vi "Draw Rect Parabolic Gradient.vi"(7 "Position":cluster{"Left":i16, "Top":i16}, 9 "Percentage(30)":dbl=30.0 format="%0.2f", 10 "Color":u32(colorbox), 11 "Size":cluster{"Width":i16, "Height":i16}) -> (3 "2D Picture":picture)   [LabVIEW 2016, in "Gradient Rectangle.lvclass"]
uses:
  Gradient Rectangle.lvclass
  <vilib>/Analysis/polynomials.llb/Scalar Polynomial Evaluation (DBL).vi
  <vilib>/Analysis/NI_AALPro.lvlib
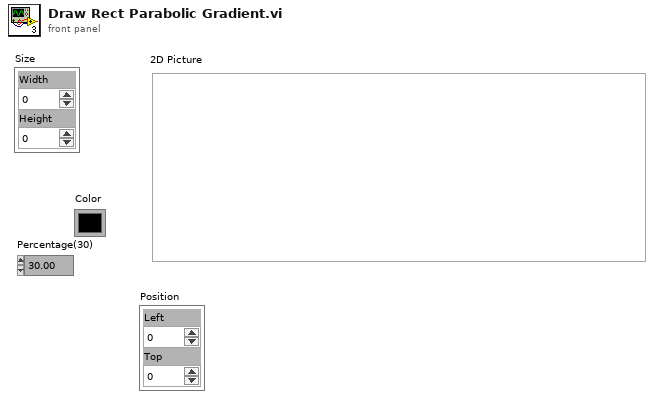
[diagram p1: front panel]
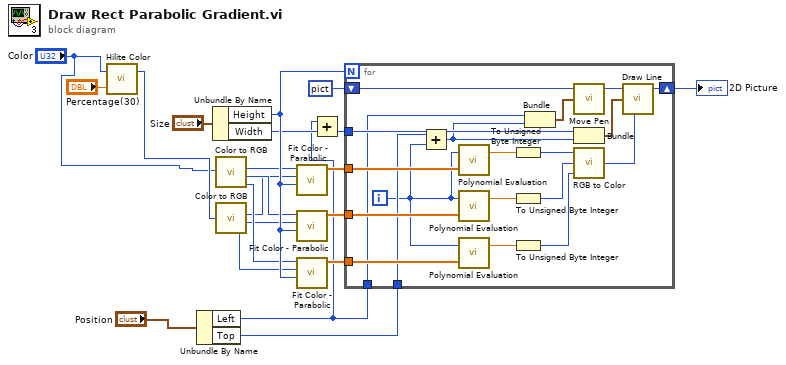
[diagram p0: block diagram]
diagram:
  n1 = call <vilib>:"Hilite Color.vi"("Percentage(30)"="Percentage(30)", "Color In"="Color") -> ("Hilite"=w6:u32)  [unwired: 1 out]
  n2 = Unbundle By Name("Position") -> ("Left"=w1:i16, "Top"=w3:i16)
  n3 = Unbundle By Name("Size") -> ("Height"=w21:i16, "Width"=w20:i16)
  n4 = call <vilib>:"Color to RGB.vi"("Color"="Color") -> ("R"=w12:u8, "G"=w15:u8, "B"=w16:u8)  [unwired: 1 out]
  n5 = call <vilib>:"Color to RGB.vi"("Color"=w6) -> ("R"=w13:u8, "G"=w14:u8, "B"=w17:u8)  [unwired: 1 out]
  n6 = call "Fit Color - Parabolic.vi"("Height"=w21, "Color Shadow"=w13, "Color Hilite"=w12) -> ("Polynomial Coefficients"=w11:dbl[])  [unwired: 8 in]
  n7 = call "Fit Color - Parabolic.vi"("Height"=w21, "Color Shadow"=w14, "Color Hilite"=w15) -> ("Polynomial Coefficients"=w18:dbl[])  [unwired: 8 in]
  n8 = call "Fit Color - Parabolic.vi"("Height"=w21, "Color Shadow"=w17, "Color Hilite"=w16) -> ("Polynomial Coefficients"=w19:dbl[])  [unwired: 8 in]
  n9 = Add(x=w1, y=w20) -> (x+y=w2:i16)
  n10 = for {
    N: w21 -> [_]
    shift-right: [w34] -> w8
    shift-left: picture data[5B] ("new picture") -> [w36]
    tunnel: w11 -> [w41]
    tunnel: w2 -> [w38]
    tunnel: w18 -> [w33]
    tunnel: w19 -> [w32]
    tunnel: w1 -> [w25]
    tunnel: w3 -> [w23]
    i -> [w22]
    n11 = Add(x=w23, y=w22) -> (x+y=w24:i32)
    n12 = call-poly <vilib>:"Polynomial Evaluation.vi"("P(x)"=w41, "a"=w22) -> ("P(a)"=w40:dbl)  [unwired: 1 out]
    n13 = call-poly <vilib>:"Polynomial Evaluation.vi"("P(x)"=w33, "a"=w22) -> ("P(a)"=w30:dbl)  [unwired: 1 out]
    n14 = call-poly <vilib>:"Polynomial Evaluation.vi"("P(x)"=w32, "a"=w22) -> ("P(a)"=w27:dbl)  [unwired: 1 out]
    n15 = To Unsigned Byte Integer(number=w40) -> (unsigned 8bit integer=w31:u8)
    n16 = To Unsigned Byte Integer(number=w30) -> (unsigned 8bit integer=w29:u8)
    n17 = To Unsigned Byte Integer(number=w27) -> (unsigned 8bit integer=w28:u8)
    n18 = Bundle("Left"=w25, w24) -> (w35:cluster{"Left":i16, i32})  [unwired: 1 in]
    n19 = call <vilib>:"Move Pen.vi"("new position"=w35, "picture"=w36) -> ("new picture"=w37:picture)  [unwired: 3 in]
    n20 = Bundle(w38, w24) -> (w39:cluster{i16, i32})  [unwired: 1 in]
    n21 = call <vilib>:"RGB to Color.vi"("B"=w28, "G"=w29, "R"=w31) -> ("Color"=w26:u32)
    n22 = call <vilib>:"Draw Line.vi"("picture"=w37, "end point"=w39, "color(black)"=w26) -> ("new picture"=w34:picture)  [unwired: 6 in]
  }
  "2D Picture" <- w8
